vi "Format condition table (SubVI).vi"(11 "file path (use dialog)":path) -> (1 "Reformated table":dbl[][](array[numeric]), 2 "Number of rows":i32, 3 "Conditions Table":string[][](array[string]))   [LabVIEW 2018]
uses:
  <vilib>/Utility/file.llb/Read Delimited Spreadsheet (string).vi
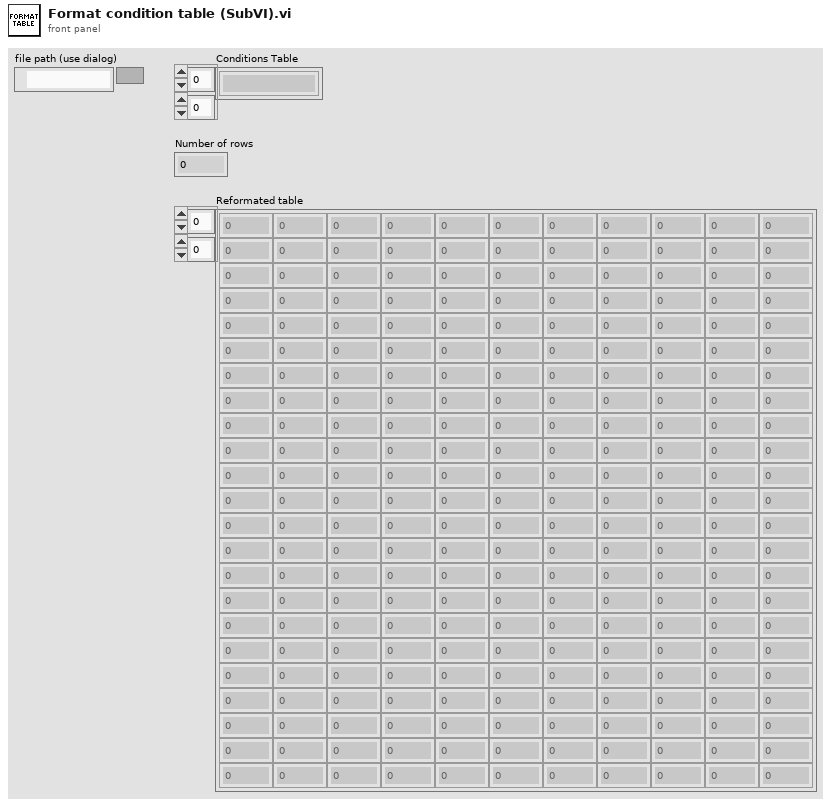
[diagram p1: front panel]
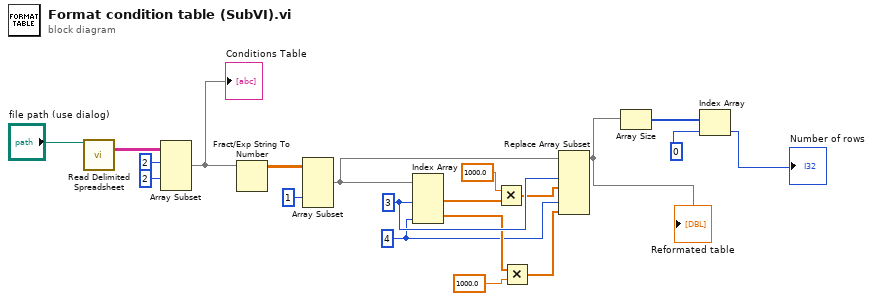
[diagram p0: block diagram]
diagram:
  w1 = 4 ("disabled index (row)")
  w20 = 3 ("index")
  n1 = call-poly <vilib>:"Read Delimited Spreadsheet.vi"("file path (dialog if empty)"="file path (use dialog)") -> ("all rows"=w11:string[][])  [unwired: 9 in, 5 out]
  n2 = Array Subset(array=w11, index (row)=2 ("index"), index (col)=2 ("index")) -> (w13:string[][])  [unwired: 2 in]
  "Conditions Table" <- w13
  n3 = Fract/Exp String To Number(string=w13) -> (number=w10:dbl[][])  [unwired: 3 in, 1 out]
  n4 = Array Subset(array=w10, index (col)=1 ("index")) -> (w16:dbl[][])  [unwired: 3 in]
  n5 = Index Array(array=w16, index (col) #1=w20, index (col) #2=w1) -> (element #1=w17:dbl[], element #2=w3:dbl[])  [unwired: 2 in]
  n6 = Multiply(x=1000.0, y=w17) -> (x*y=w18:dbl[])
  n7 = Multiply(x=w3, y=1000.0) -> (x*y=w2:dbl[])
  n8 = Replace Array Subset(array=w16, new element #1=w18, index (col) #1=w20, new element #2=w2, index (col) #2=w1) -> (w19:dbl[][])  [unwired: 2 in]
  "Reformated table" <- w19
  n9 = Array Size(array=w19) -> (size(s)=w7:i32[])
  n10 = Index Array(array=w7, index=0) -> (element=→"Number of rows":i32)
